vi "test - Cluster Changed with Leaf Element Name.vi"(8 "error in (no error)":errorcluster, 11 "TestCase in":refnum<class "testcase-Supported-Datatype.lvclass">) -> (0 "error out":errorcluster, 3 "TestCase out":refnum<class "testcase-Supported-Datatype.lvclass">)   [LabVIEW 2017, in "testcase-Supported-Datatype.lvclass"]
uses:
  testcase-Supported-Datatype.lvclass
  bb895ddf-ce8c-494e-8883-52f08cc6326c.vi
  280d6c91-db87-4815-9f1c-5b2cc9a3a532.vi
  75061575-983a-4300-85c5-60252db20c2a.vi
  addons/API-String-Arugments-Support/_Support/Convert API String Arguments to Data(variant).vi
  <vilib>/addons/_JKI Toolkits/VI Tester/TestCase.llb/TestCase.lvclass
  C:/Program Files (x86)/National Instruments/LabVIEW 2017/vi.lib/addons/_JKI Toolkits/VI Tester/TestCase.llb/TestCase.lvclass
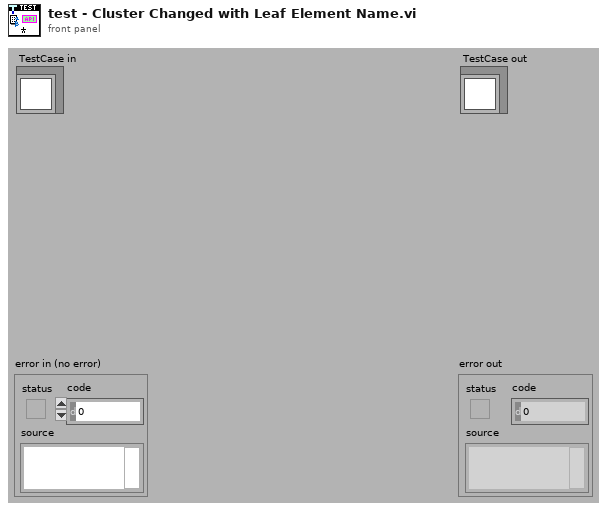
[diagram p1: front panel]
types:
  T1 = cluster{"grade":string, "Child1":cluster{"class":string, "Child1-2":cluster{"Name":string}}, "Bool":bool}
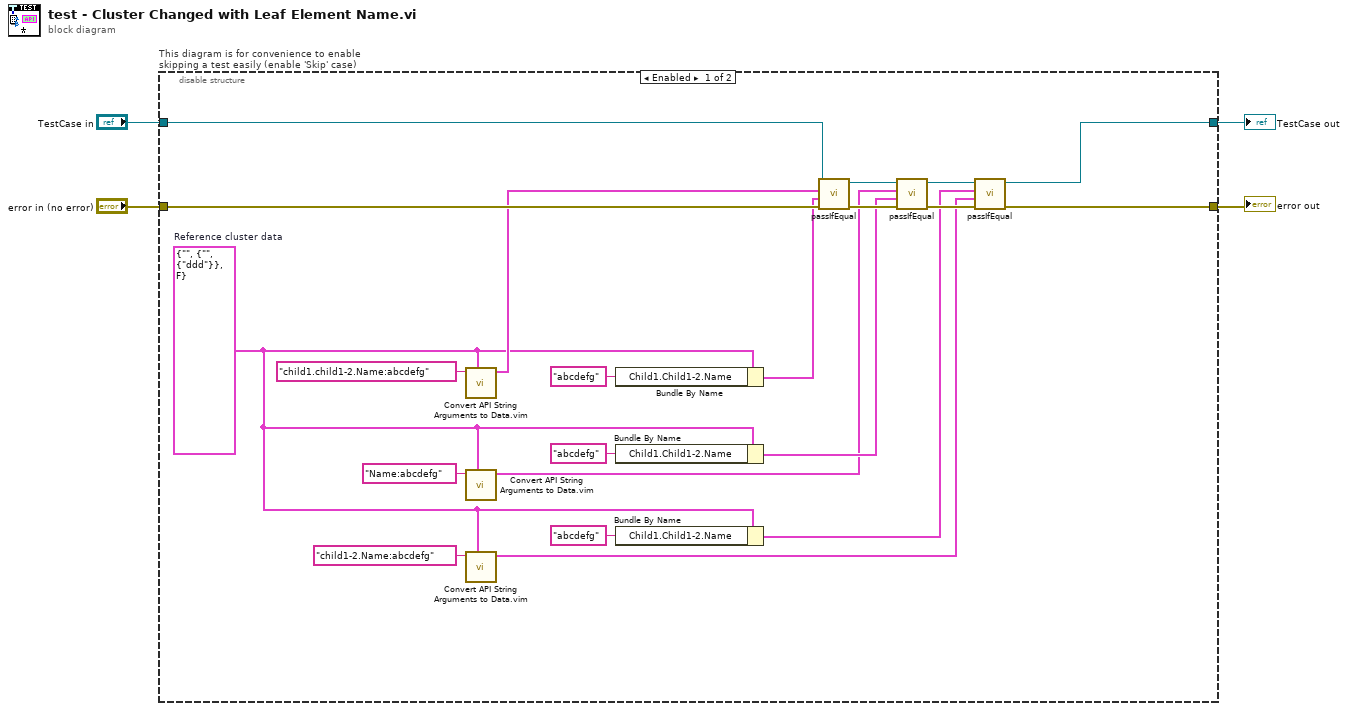
[diagram p0: block diagram]
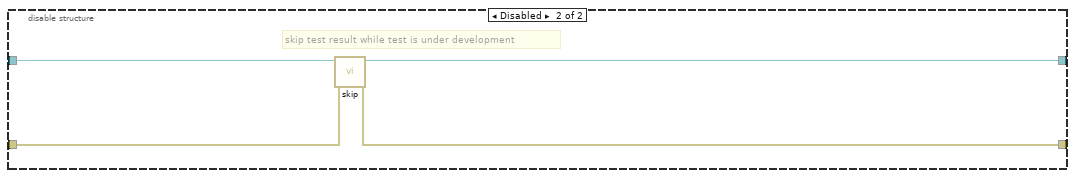
[diagram p2: hidden frame]
diagram:
  n1 = disable-structure "This diagram is for convenience to enable skipping a test easily (enable 'Skip' case)" shown="Enabled" {
    disable-tunnel: "TestCase in" -> [w24 w29]
    disable-tunnel: [w5 w27] -> w1
    disable-tunnel: [w6 w28] -> w3
    disable-tunnel: "error in (no error)" -> [w20 w26]
    frame Enabled {
      w9 = T1 {"grade"="", "Child1"={"class"="", "Child1-2"={"Name"="ddd"}}, "Bool"=FALSE}  # Reference cluster data
      n2 = call "Convert API String Arguments to Data.vim"("Reference Type"=w9, "API String"="child1.child1-2.Name:abcdefg" ("String")) -> ("Data"=w16:T1)  [unwired: 6 in, 1 out]
      n3 = call "Convert API String Arguments to Data.vim"("Reference Type"=w9, "API String"="Name:abcdefg" ("String")) -> ("Data"=w12:T1)  [unwired: 6 in, 1 out]
      n4 = call "Convert API String Arguments to Data.vim"("Reference Type"=w9, "API String"="child1-2.Name:abcdefg" ("String")) -> ("Data"=w7:T1)  [unwired: 6 in, 1 out]
      n5 = Bundle By Name(cluster=w9, "Child1.Child1-2.Name"="abcdefg") -> (w17:T1)
      n6 = Bundle By Name(cluster=w9, "Child1.Child1-2.Name"="abcdefg") -> (w13:T1)
      n7 = Bundle By Name(cluster=w9, "Child1.Child1-2.Name"="abcdefg") -> (w8:T1)
      n8 = call-dynamic "passIfEqual.vi"("error in (no error)"=w20, "y"=w17, "x"=w16, "TestCase in"=w24) -> ("error out"=w25:errorcluster, "TestCase out"=w23:refnum<class "testcase-Supported-Datatype.lvclass">)  [unwired: 6 in]
      n9 = call-dynamic "passIfEqual.vi"("error in (no error)"=w25, "y"=w13, "x"=w12, "TestCase in"=w23) -> ("error out"=w21:errorcluster, "TestCase out"=w22:refnum<class "testcase-Supported-Datatype.lvclass">)  [unwired: 6 in]
      n10 = call-dynamic "passIfEqual.vi"("error in (no error)"=w21, "y"=w7, "x"=w8, "TestCase in"=w22) -> ("error out"=w6:errorcluster, "TestCase out"=w5:refnum<class "testcase-Supported-Datatype.lvclass">)  [unwired: 6 in]
    }
    frame Disabled {
      # "skip test result while test is under development"
      n11 = call <vilib>:"skip.vi"("error in (no error)"=w26, "TestCase in"=w29) -> ("error out"=w28:errorcluster, "TestCase out"=w27:refnum<class "testcase-Supported-Datatype.lvclass">)  [unwired: 8 in]
    }
  }
  "error out" <- w3
  "TestCase out" <- w1
